vi "Get COB.vi"(8 "error in":errorcluster, 11 "PDO Slot in":refnum<class "PDO Slot.lvclass">) -> (0 "error out":errorcluster, 2 "COB-ID":u32 format="%.0x", 3 "PDO Slot out":refnum<class "PDO Slot.lvclass">)   [LabVIEW 2019, in "PDO Grid.lvlib" / "PDO Slot.lvclass"]
uses:
  PDO Slot.lvclass
  PDO Slot.lvclass/PDO Slot.ctl
  Core/PDO Communication Parameter/PDO Communication Parameter.lvclass/PDO Communication Parameter.ctl
  Core/PDO Communication Parameter/PDO Communication Parameter.lvclass
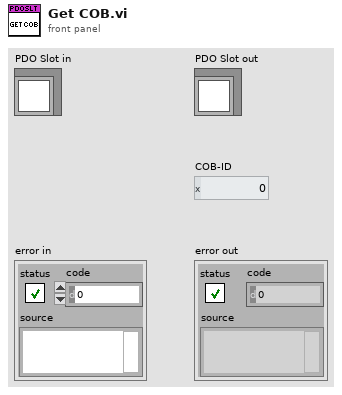
[diagram p1: front panel]
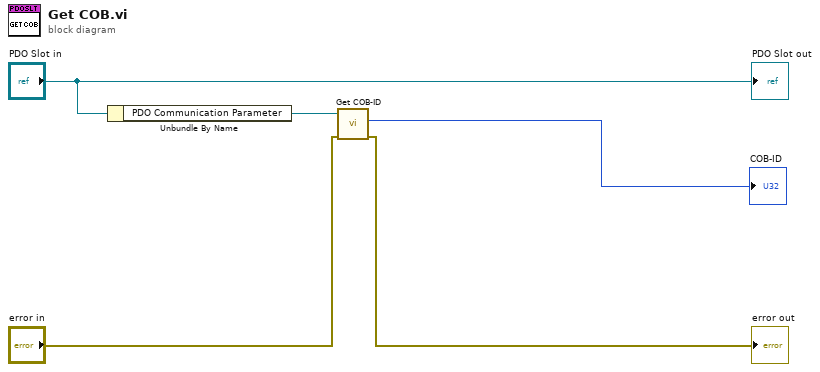
[diagram p0: block diagram]
diagram:
  n1 = Unbundle By Name("PDO Slot in") -> ("PDO Communication Parameter"=w4:refnum<class "PDO Communication Parameter.lvclass">)
  n2 = call "Get COB-ID.vi"("error in (no error)"="error in", "PDO Communication Parameter in"=w4) -> ("error out"=→"error out":errorcluster, "COB-ID"=→"COB-ID":u32)  [unwired: 7 in, 1 out]
  "PDO Slot out" <- "PDO Slot in"
